vi "Initialize.vi"(8 "error in":errorcluster, 11 "Plugin in":refnum<class "Sequencer with Output Values.lvclass">) -> (0 "error out":errorcluster, 3 "Plugin out":refnum<class "Sequencer with Output Values.lvclass">)   [LabVIEW 2024, in "Sequencer with Output Values.lvlib" / "Sequencer with Output Values.lvclass"]
uses:
  Sequencer with Output Values.lvclass
  C:/Program Files/National Instruments/LabVIEW 2024/vi.lib/FlexLogger/SDK/PluginSDK.lvlibp/PEFClasses/SDK/Plugin/Plugin.lvclass
  <vilib>/FlexLogger/SDK/PluginSDK.lvlibp/PEFClasses/SDK/Processing Element/Timing Parameters.ctl
  <vilib>/FlexLogger/SDK/PluginSDK.lvlibp/PEFClasses/SDK/Processing Element/Timing Method.ctl
  Params.ctl
  Step Settings.ctl
  Sequencer with Output Values.lvclass/Sequencer with Output Values.ctl
  <vilib>/FlexLogger/SDK/PluginSDK.lvlibp/PEFClasses/SDK/Producer Channel/Producer Channel.lvclass
  C:/Program Files/National Instruments/LabVIEW 2024/vi.lib/FlexLogger/SDK/PluginSDK.lvlibp/PEFClasses/SDK/Channel/Channel.lvclass
  <vilib>/FlexLogger/SDK/PluginSDK.lvlibp/PEFClasses/SDK/Producer Channel/Create Producer Channel.vi
  Global Strings.vi
  <vilib>/FlexLogger/SDK/PluginSDK.lvlibp/PEFClasses/SDK/Plugin/ParameterAccess/Write Boolean.vi
  <vilib>/FlexLogger/SDK/PluginSDK.lvlibp/PEFClasses/SDK/Plugin/ParameterAccess/Write DBL.vi
  <vilib>/FlexLogger/SDK/PluginSDK.lvlibp/PEFClasses/SDK/Plugin/ParameterAccess/Write I32.vi
  <vilib>/FlexLogger/SDK/PluginSDK.lvlibp/PEFClasses/SDK/Plugin/Plugin.lvclass
  <vilib>/FlexLogger/SDK/PluginSDK.lvlibp/PEFClasses/SDK/Processing Element/Processing Element.lvclass
  <vilib>/FlexLogger/SDK/PluginSDK.lvlibp
  C:/Program Files/National Instruments/LabVIEW 2024/vi.lib/FlexLogger/SDK/PluginSDK.lvlibp/PEFClasses/SDK/Processing Element/Processing Element.lvclass
  C:/dev/niflexlogger-plugins/plugins/Sequencer with Output Values/source/Sequencer with Output Values/Sequencer with Output Values.lvclass
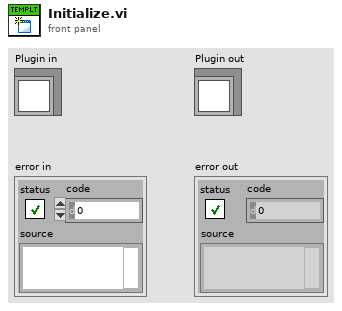
[diagram p1: front panel]
types:
  T1 = typedef "Step Settings.ctl" = cluster{"Duration":dbl, "Mode":string, "Delay Between Values":dbl, "Analog Values":string[], "Digital Values":string[]}
  T2 = typedef "Sequencer with Output Values.lvlib/Sequencer with Output Values.lvclass/Params.ctl" = cluster{"Step Values":T1[], "Only Execute When Test Running":bool, "Current Sequence ID":u32, "Total Iterations":u32, "Last Timestamp":timestamp, "Number of Sequence Steps":i32, "Number of Analog Channels":i32, "Number of Digital Channels":i32, "Delay Before Starting Sequence":dbl}
  T3 = typedef "PluginSDK.lvlibp/Processing Element.lvclass/Timing Parameters.ctl" = cluster{"Timing Method":T4, "Timing Period (ms)":i32}
  T4 = typedef "PluginSDK.lvlibp/Processing Element.lvclass/Timing Method.ctl" = enum16{"Periodic", "Immediate", "On Data Ready", "Triggered"}
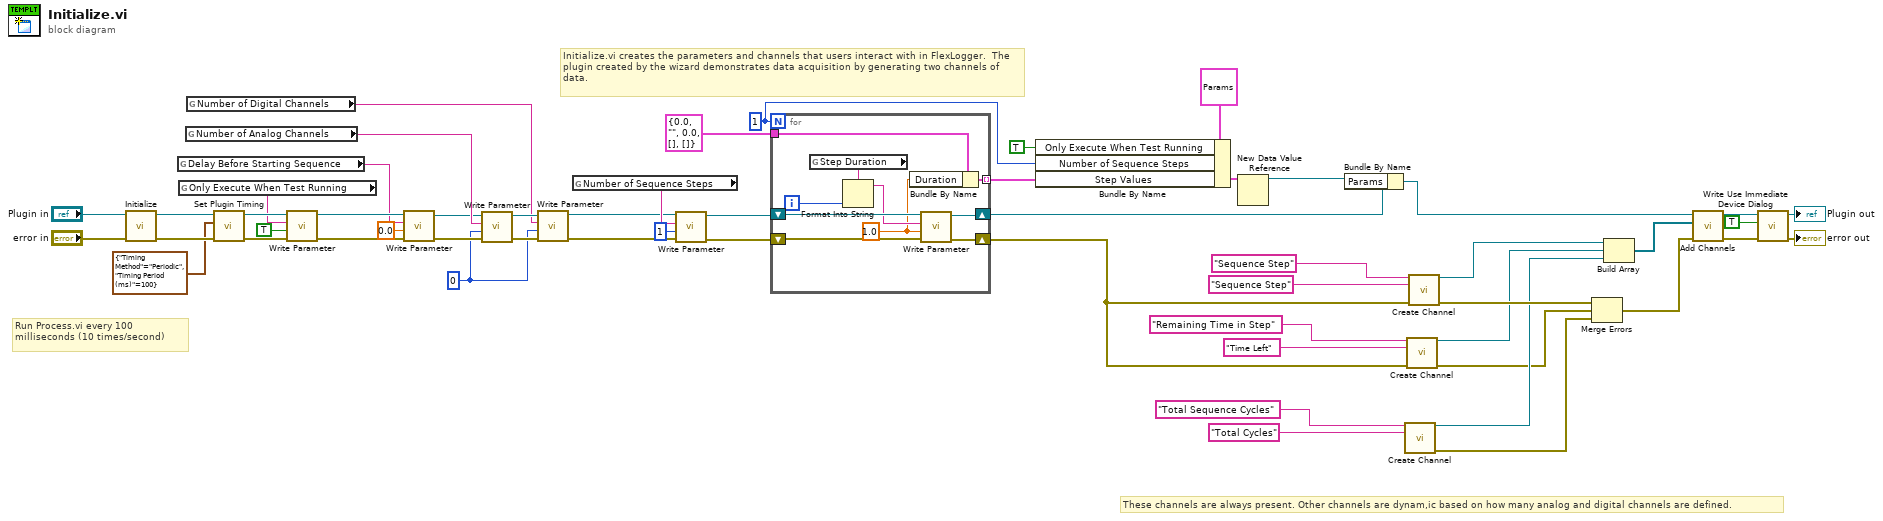
[diagram p0: block diagram]
diagram:
  w13 = 0 ("Value")
  w37 = 1
  # "These channels are always present. Other channels are dynam,ic based on how many analog and digital channels are defined."
  # "Run Process.vi every 100 milliseconds (10 times/second)"
  # "Initialize.vi creates the parameters and channels that users interact with in FlexLogger.  The plugin created by the wizard demonstrates data acquisition by generating two channels of data."
  n1 = call-parent "Initialize.vi"("error in (no error)"="error in", "Plugin in"="Plugin in") -> ("error out"=w53:errorcluster, "Plugin out"=w51:refnum<class "Sequencer with Output Values.lvclass">)  [unwired: 8 in]
  n2 = global read "Global Strings.vi" "Delay Before Starting Sequence"() -> (w21:string)
  n3 = global read "Global Strings.vi" "Only Execute When Test Running"() -> (w25:string)
  n4 = global read "Global Strings.vi" "Number of Analog Channels"() -> (w19:string)
  n5 = global read "Global Strings.vi" "Number of Digital Channels"() -> (w14:string)
  n6 = call <vilib>:"Set Plugin Timing.vi"("error in (no error)"=w53, "Timing Parameters"=T3 {"Timing Method"=enum."Periodic", "Timing Period (ms)"=100}, "Plugin in"=w51) -> ("error out"=w47:errorcluster, "Plugin out"=w48:refnum<class "Sequencer with Output Values.lvclass">)  [unwired: 7 in]
  n7 = call-poly <vilib>:"Write Parameter.vi"("error in (no error)"=w47, "Value"=TRUE, "Name"=w25, "Plugin in"=w48) -> ("error out"=w22:errorcluster, "Plugin out"=w23:refnum<class "Sequencer with Output Values.lvclass">)  [unwired: 6 in]
  n8 = call-poly <vilib>:"Write Parameter.vi"("error in (no error)"=w22, "Value"=0.0, "Name"=w21, "Plugin in"=w23) -> ("error out"=w17:errorcluster, "Plugin out"=w18:refnum<class "Sequencer with Output Values.lvclass">)  [unwired: 6 in]
  n9 = call-poly <vilib>:"Write Parameter.vi"("error in (no error)"=w17, "Value"=w13, "Name"=w19, "Plugin in"=w18) -> ("error out"=w15:errorcluster, "Plugin out"=w16:refnum<class "Sequencer with Output Values.lvclass">)  [unwired: 6 in]
  n10 = call-poly <vilib>:"Write Parameter.vi"("error in (no error)"=w15, "Value"=w13, "Name"=w14, "Plugin in"=w16) -> ("error out"=w11:errorcluster, "Plugin out"=w12:refnum<class "Sequencer with Output Values.lvclass">)  [unwired: 6 in]
  n11 = global read "Global Strings.vi" "Number of Sequence Steps"() -> (w24:string)
  n12 = call-poly <vilib>:"Write Parameter.vi"("error in (no error)"=w11, "Value"=1, "Name"=w24, "Plugin in"=w12) -> ("error out"=w38:errorcluster, "Plugin out"=w39:refnum<class "Sequencer with Output Values.lvclass">)  [unwired: 6 in]
  n13 = for {
    N: w37 -> [_]
    shift-right: [w62] -> w45
    shift-left: w39 -> [w65]
    shift-right: [w61] -> w8
    shift-left: w38 -> [w64]
    tunnel: T1 {"Duration"=0.0, "Mode"="", "Delay Between Values"=0.0, "Analog Values"=[], "Digital Values"=[]} -> [w58]
    tunnel: [w56] -> w1 mode=indexing
    i -> [w60]
    w57 = 1.0 ("Value")
    n14 = global read "Global Strings.vi" "Step Duration"() -> (w59:string)
    n15 = Format Into String(format string=w59, w60) -> (resulting string=w63:string)  [unwired: 2 in, 1 out]
    n16 = Bundle By Name(cluster=w58, "Duration"=w57) -> (w56:T1)
    n17 = call-poly <vilib>:"Write Parameter.vi"("error in (no error)"=w64, "Value"=w57, "Name"=w63, "Plugin in"=w65) -> ("error out"=w61:errorcluster, "Plugin out"=w62:refnum<class "Sequencer with Output Values.lvclass">)  [unwired: 6 in]
  }
  n18 = Bundle By Name(cluster=T2 {"Step Values"=[], "Only Execute When Test Running"=TRUE, "Current Sequence ID"=0, "Total Iterations"=0, "Last Timestamp"=timestamp(0 s since 1904-01-01), "Number of Sequence Steps"=0, "Number of Analog Channels"=0, "Number of Digital Channels"=0, "Delay Before Starting Sequence"=0.0}, "Only Execute When Test Running"=TRUE, "Number of Sequence Steps"=w37, "Step Values"=w1) -> (w43:T2)
  n19 = New Data Value Reference(data value=w43) -> (data value reference=w41:refnum<data-value>)  [unwired: 1 in, 1 out]
  n20 = Bundle By Name(cluster=w45, "Params"=w41) -> (w42:refnum<class "Sequencer with Output Values.lvclass">)
  n21 = call-poly <vilib>:"Create Channel.vi"("Unique Channel Identifier"="Total Sequence Cycles" ("format string"), "Default Channel Name"="Total Cycles" ("format string")) -> ("Producer Channel"=w6:refnum<class "Producer Channel.lvclass">, "error out"=w4:errorcluster)  [unwired: 12 in]
  n22 = call-poly <vilib>:"Create Channel.vi"("Unique Channel Identifier"="Remaining Time in Step" ("format string"), "Default Channel Name"="Time Left" ("format string"), "error in (no error)"=w8) -> ("Producer Channel"=w7:refnum<class "Producer Channel.lvclass">, "error out"=w5:errorcluster)  [unwired: 11 in]
  n23 = call-poly <vilib>:"Create Channel.vi"("Unique Channel Identifier"="Sequence Step" ("format string"), "Default Channel Name"="Sequence Step" ("format string"), "error in (no error)"=w8) -> ("Producer Channel"=w28:refnum<class "Producer Channel.lvclass">, "error out"=w29:errorcluster)  [unwired: 11 in]
  n24 = Merge Errors(w29, w5, w4) -> (w49:errorcluster)
  n25 = Build Array(w28, w7, w6) -> (w50:refnum<class "Producer Channel.lvclass">[])
  n26 = call <vilib>:"Add Channels.vi"("error in (no error)"=w49, "Channels"=w50, "Plugin in"=w42) -> ("error out"=w35:errorcluster, "Plugin out"=w36:refnum<class "Sequencer with Output Values.lvclass">)  [unwired: 7 in]
  n27 = call <vilib>:"Write Use Immediate Device Dialog.vi"("error in (no error)"=w35, "Use Immediate Device Dialog?"=TRUE, "Plugin in"=w36) -> ("error out"=→"error out":errorcluster, "Plugin out"=→"Plugin out":refnum<class "Sequencer with Output Values.lvclass">)  [unwired: 7 in]
